vi "KillModalVIs.vi"() -> ()   [LabVIEW 2020]
doc: "Utility to close a modal VI when it has been brought to the foreground and reserved to run. This locks up LabVIEW so this VI will present a list of VIs to optionally close.\nScott Hannahs, National High Magnetic Field Lab\nJanuary 2005\n<sth@magnet.fsu.edu>"
panel:
  in  "OK Button":bool
  in  "VIs to close":i32[](listbox)=[0]
  out "Slide":i32(slide)
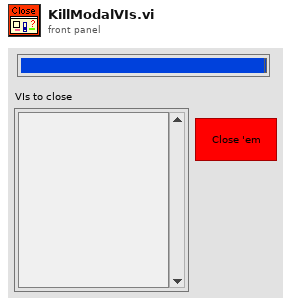
[diagram p1: front panel]
types:
  T1 = enum32{"Bad", "Idle", "Run top level", "Running"}
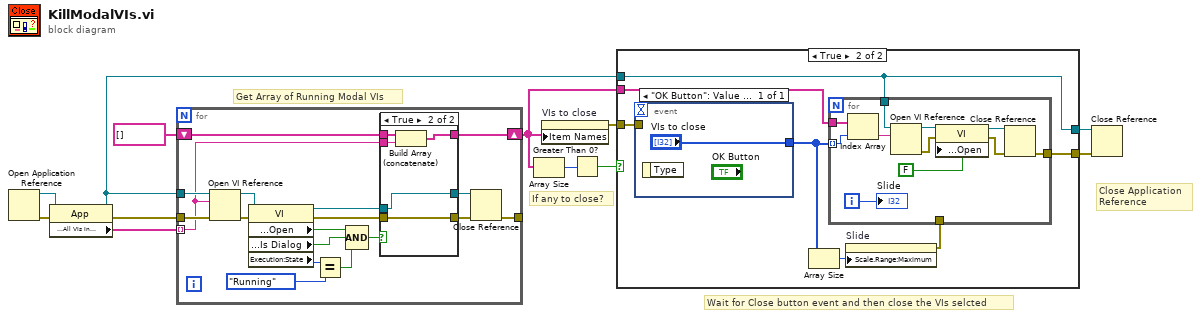
[diagram p0: block diagram]
diagram:
  # "If any to close?"
  # "Close Application\nReference"
  # "Wait for Close button event and then close the VIs selcted"
  # "Get Array of Running Modal VIs"
  n1 = Open Application Reference() -> (0:w12:errorcluster, 3:w11:refnum<vi>)  [unwired: 4 in]
  n2 = property class="App"(reference=w11, error in=w12) -> (reference out=w2:refnum<vi>, error out=w10:errorcluster, "Application:All VIs In Memory"=w9:string[])
  n3 = for {
    tunnel: w10 -> [w30]
    tunnel: w9 -> [w14] mode=indexing
    tunnel: w2 -> [w15]
    tunnel: [w19] -> _
    shift-right: [w13] -> w5
    shift-left: string[] [] -> [w16]
    n4 = Open VI Reference(application reference (local)=w15, vi path=w14, error in (no error)=w30) -> (vi reference=w28:refnum<vi>, error out=w29:errorcluster)  [unwired: 3 in]
    n5 = property class="VI"(reference=w28, error in=w29) -> (reference out=w22:refnum<vi>, error out=w23:errorcluster, "Front Panel Window:Open"=w25:bool, "Front Panel Window:Is Dialog"=w26:bool, "Execution:State"=w27:T1)
    n6 = Equal?(x=w27, y=T1."Running") -> (x = y?=w17:bool)
    n7 = Compound Arithmetic op=AND(w25, w26, w17) -> (w24:bool)
    n8 = case shown="True" w24 {
      tunnel: w23 -> [w32 w36]
      tunnel: w22 -> [w33 w34]
      tunnel: [w32 w36] -> w21
      tunnel: [w33 w34] -> w20
      tunnel: w16 -> [w31 w38]
      tunnel: w14 -> [_ w37]
      tunnel: [w31 w35] -> w13
      frame False {
      }
      frame True {
        n9 = Build Array (concatenate)(w38, w37) -> (w35:string[])
      }
    }
    n10 = Close Reference(reference=w20, error in (no error)=w21) -> (error out=w19:errorcluster)
  }
  n11 = Array Size(array=w5) -> (size(s)=w4:i32)
  n12 = property on="VIs to close" class="LstBox (strict)"("Item Names"=w5) -> (error out=w7:errorcluster)  [unwired: 2 in, 1 out]
  n13 = Greater Than 0?(x=w4) -> (x > 0?=w3:bool)
  n14 = case shown="True" w3 {
    tunnel: w7 -> [w40 w46]
    tunnel: [w40 w43] -> w6
    tunnel: w5 -> [_ w42]
    tunnel: w2 -> [w39 w41]
    tunnel: [w39 w41] -> w1
    frame False {
    }
    frame True {
      n15 = event shown="[0] \"OK Button\": Value Change" {
        selector: _ -> [_]
        dyn-events: _ -> [_]
        timeout: _ -> [_]
        tunnel: w46 -> [_]
        tunnel: ["VIs to close"] -> w45
        event "OK Button": Value Change {
          n16 = event-data() -> ()  [unwired: 1 in, 1 out]
        }
      }
      n17 = Array Size(array=w45) -> (size(s)=w47:i32)
      n18 = property on="Slide" class="Slide (strict)"("Scale.Range:Maximum"=w47) -> (error out=w44:errorcluster)  [unwired: 2 in, 1 out]
      n19 = for {
        tunnel: w45 -> [w55] mode=indexing
        tunnel: w44 -> [_]
        tunnel: w42 -> [w56]
        tunnel: w41 -> [w49]
        tunnel: [w48] -> w43
        i -> [w58]
        n20 = Index Array(array=w56, index=w55) -> (element=w57:string)
        n21 = Open VI Reference(application reference (local)=w49, vi path=w57) -> (vi reference=w54:refnum<vi>, error out=w53:errorcluster)  [unwired: 4 in]
        n22 = property class="VI"(reference=w54, error in=w53, "Front Panel Window:Open"=FALSE) -> (reference out=w51:refnum<vi>, error out=w50:errorcluster)
        n23 = Close Reference(reference=w51, error in (no error)=w50) -> (error out=w48:errorcluster)
        "Slide" <- w58
      }
    }
  }
  n24 = Close Reference(reference=w1, error in (no error)=w6) -> ()  [unwired: 1 out]
